vi "AlliGator Compute Smoothed Complex Phasor Array.vi"(8 "error in (no error)":errorcluster, 9 "Time-Gated Reference Decay":cluster{"t Array":dbl[], "I Array":dbl[]}, 10 "Image Array":T17[](array[typedef]), 11 "Sum Image":T17) -> (0 "error out":errorcluster, 1 "Phasor Plot Parameters":T1={"Phasor Frequency"=0.0, "Decay Preprocessing Options & Parameters"={"Background Subtraction Parameters"={"Background Definition Range"={"Min Gate"=0.0, "Max Gate"=0.0}, "Baseline Subtraction Method"=enum."Mean", "Background Subtraction?"=FALSE, "Background File"=path "", "Background Constant"=0.0, "Background Scaling Factor"=1.0, "Background Pile-up Correction"=FALSE, "Background Pixel Well Capacity"=1}, "Decay Preprocessing Parameters"={"Background Subtraction"=FALSE, "Straighten Decay"=FALSE, "Reverse Gates"=FALSE, "1-Normalized Decay"=FALSE, "Smoothen Decay"=FALSE, "Smoothing Parameter"=0.0, "Shift Decay"=FALSE, "Decay Shift Parameters"={"Type"=enum."Default", "Shift"=0.0, "Threshold"=0.0, "Rotate"=FALSE}, "Extrapolate Decay"=FALSE, "Additional Points"=0, "Head Fraction"=0.0, "Pixel-Normalize Decay"=FALSE, "Use Periodicity"=FALSE, "Use Cursors"=FALSE, "Tail Fraction"=0.0, "Use Decay Pre-Processing"=TRUE, "Fold Decay"=FALSE, "# Folds"=1, "[0-1]-Normalized Decay"=FALSE}, "Preprocessing Steps Order"=[]}, "FLI Dataset Modified"=FALSE, "Source Image Settings"={"Low Count Pixels Rejection Options"={"Background Low Threshold Factor"=0.0, "Fixed Low Background Threshold"=0.0, "Reject Low Count Pixels"=FALSE, "Low Percentile"=0.0}, "High Count Pixels Rejection Options"={"Background High Threshold Factor"=0.0, "Fixed High Background Threshold"=20000.0, "Reject High Count Pixels"=FALSE, "High Percentile"=100.0}}, "Data Information"={"Gate Width"=0.0, "Gate Separation"=0.0, "Step (Gate Separation)"=0, "Laser Period"=0.0, "SYNC Period"=0.0, "Channel Name"=0, "Channel Arithmetic"=enum."None", "Pile-up Correction"=FALSE, "Pixel Well Capacity"=1, "Dataset Scaling Factor"=1.0}, "Phasor Plot"={"Phasor Plot Smoothing Options"={"Use Phasor Plot Smoothing"=FALSE, "Kernel Type"=enum."Uniform", "Bin"=1, "Algorithm"=enum."Rapid"}, "Phasor Plot Size"={"H"=0, "V"=0, "Margin"=0.0}, "Selected Image ROI(s)"=FALSE, "All Image ROIs"=FALSE, "Selected Source Image ROI"=0, "Source Image ROIs"=[]}} {"Phasor Plot"."Source Image ROIs"."ROI Descriptor"."Contours"."Type" items=["No Selection", "Point", "Line", "Rectangle", "Oval", "Polygon", "Freehand Region", "Annulus", "Unused2", "Unused3", "Broken Line", "Freehand Line", "Rotated Rectangle"]; "Phasor Plot"."Phasor Plot Smoothing Options"."Bin" min=1 step=2; "Data Information"."Dataset Scaling Factor" min=0.0; "Data Information"."Pixel Well Capacity" min=1 step=1; "Data Information"."Channel Name" items=["Gate"]; "Source Image Settings"."High Count Pixels Rejection Options"."High Percentile" min=0.0 max=100.0; "Source Image Settings"."Low Count Pixels Rejection Options"."Low Percentile" min=0.0 max=100.0; "Decay Preprocessing Options & Parameters"."Decay Preprocessing Parameters"."# Folds" min=1; "Decay Preprocessing Options & Parameters"."Background Subtraction Parameters"."Background Pixel Well Capacity" min=1 step=1}, 2 "Corrected Complex Phasor Array out (VxH)":csg[][](array[numeric]), 3 "Valid Pixel?":bool[][](array[boolean]), 4 "Message":string, 5 "Pre-processed Sum Image (V x H)":sgl[][](array[numeric]), 6 "Phasor Array updated":bool)   [LabVIEW 2021, in "AlliGator Phasor Plot.lvlib"]
doc: "Computes the (smoothed) array of single-pixel phasors."
uses:
  AlliGator Phasor Plot.lvlib
  <vilib>/vision/Image Controls.llb/IMAQ Image.ctl
  AlliGator Phasor Plot Parameters v2.ctl
  Decay Analysis/Decay Preprocessing/AlliGator Decay Preprocessing Options.ctl
  Decay Analysis/Decay Preprocessing/AlliGator Background Subtraction Parameters.ctl
  Decay Analysis/Decay Preprocessing/AlliGator Baseline Subtraction Method.ctl
  Decay Analysis/Decay Preprocessing/AlliGator Decay Preprocessing Parameters.ctl
  Graphs/XY Graph/XY Graph Plot Shift Parameters.ctl
  Graphs/XY Graph/XY Graph Plot Shift Method.ctl
  Settings/AlliGator Low Count Pixels Rejection Options.ctl
  Settings/AlliGator High Count Pixels Rejection Options.ctl
  Settings/AlliGator Gate Arithmetic.ctl
  AlliGator Phasor Plot Smoothing Options.ctl
  Arrays/Kernel Type.ctl
  Arrays/Smoothing Algorithm.ctl
  AlliGator Phasor Plot Size.ctl
  Image/Named ROI Description.ctl
  Globals, Variables, Constants/AlliGator Variables List.ctl
  Settings/AlliGator Pixel Counts Constraints.ctl
  Phasor/Phasor.lvlib
  Decay Analysis/Decay Processing/AlliGator Decay Processing.lvlib
  Globals, Variables, Constants/AlliGator Globals, Variables & Constants.lvlib
  Settings/AlliGator Settings.lvlib
  Decay Analysis/Decay Preprocessing/AlliGator Decay Preprocessing.lvlib
  Graphs/XY Graph/XY Graph Add-Ons.lvlib
  Arrays/Arrays.lvlib
  Image/Image.lvlib
panel:
  # "see the AlliGator License on the block diagram (Ctrl+E or Window:Show Block Diagram)"
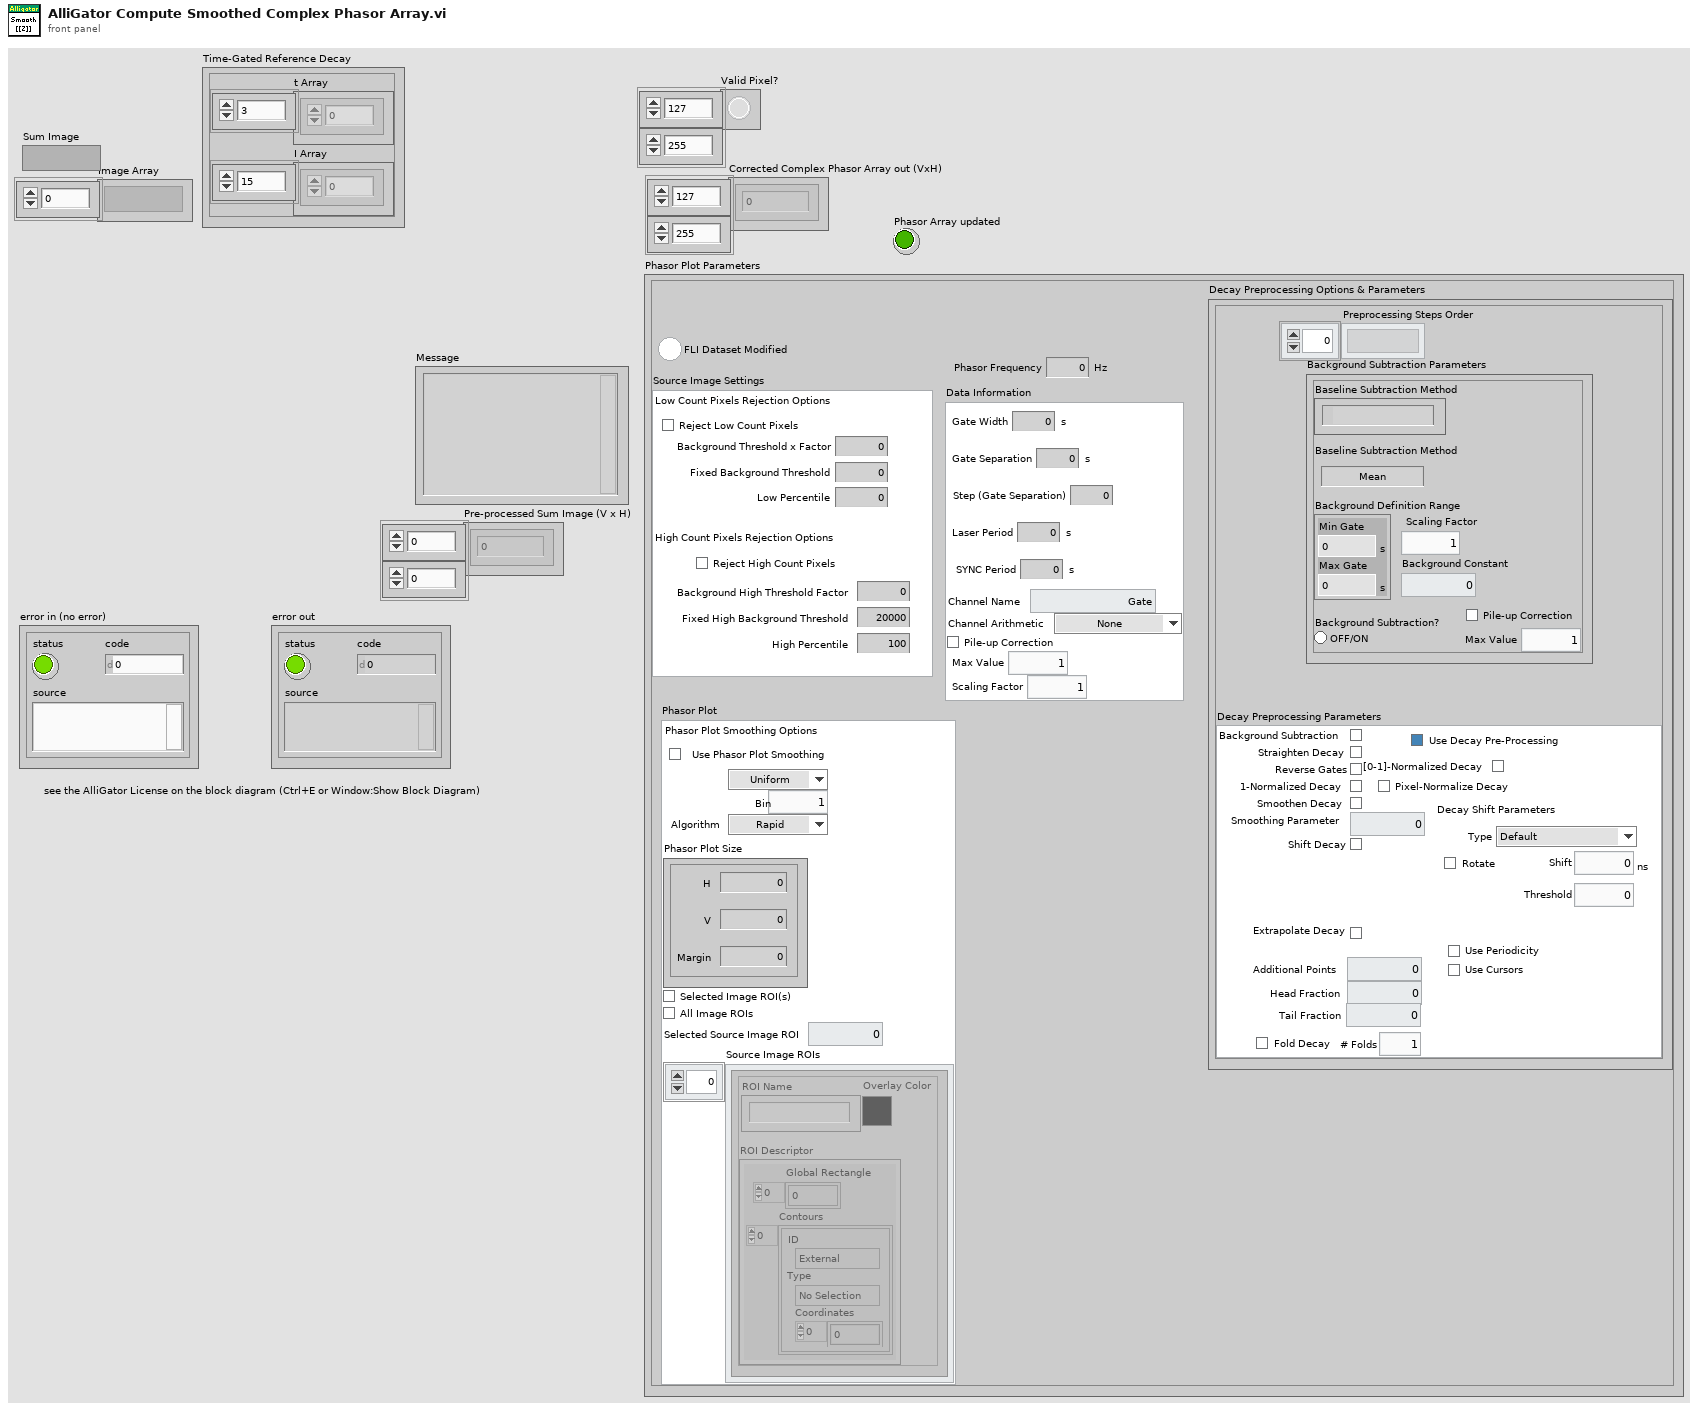
[diagram p1: front panel]
types:
  T1 = typedef "AlliGator Phasor Plot.lvlib/AlliGator Phasor Plot Parameters v2.ctl" = cluster{"Phasor Frequency":dbl[unit], "Decay Preprocessing Options & Parameters":T2, "FLI Dataset Modified":bool, "Source Image Settings":cluster{"Low Count Pixels Rejection Options":T8, "High Count Pixels Rejection Options":T9}, "Data Information":cluster{"Gate Width":dbl[unit], "Gate Separation":dbl[unit], "Step (Gate Separation)":i32, "Laser Period":dbl[unit], "SYNC Period":dbl[unit], "Channel Name":u16, "Channel Arithmetic":T10, "Pile-up Correction":bool, "Pixel Well Capacity":u32, "Dataset Scaling Factor":dbl}, "Phasor Plot":cluster{"Phasor Plot Smoothing Options":T11, "Phasor Plot Size":T14, "Selected Image ROI(s)":bool, "All Image ROIs":bool, "Selected Source Image ROI":i32, "Source Image ROIs":T15[]}}
  T2 = typedef "AlliGator Decay Preprocessing.lvlib/AlliGator Decay Preprocessing Options.ctl" = cluster{"Background Subtraction Parameters":T3, "Decay Preprocessing Parameters":T5, "Preprocessing Steps Order":string[]}
  T3 = typedef "AlliGator Decay Preprocessing.lvlib/AlliGator Background Subtraction Parameters.ctl" = cluster{"Background Definition Range":cluster{"Min Gate":dbl[unit], "Max Gate":dbl[unit]}, "Baseline Subtraction Method":T4, "Background Subtraction?":bool, "Background File":path, "Background Constant":dbl, "Background Scaling Factor":dbl, "Background Pile-up Correction":bool, "Background Pixel Well Capacity":u32}
  T4 = typedef "AlliGator Decay Preprocessing.lvlib/AlliGator Baseline Subtraction Method.ctl" = enum16{"Mean", "Min", "Square Gated Single-Exponential", "File", "Constant"}
  T5 = typedef "AlliGator Decay Preprocessing.lvlib/AlliGator Decay Preprocessing Parameters.ctl" = cluster{"Background Subtraction":bool, "Straighten Decay":bool, "Reverse Gates":bool, "1-Normalized Decay":bool, "Smoothen Decay":bool, "Smoothing Parameter":dbl, "Shift Decay":bool, "Decay Shift Parameters":T6, "Extrapolate Decay":bool, "Additional Points":u32, "Head Fraction":dbl, "Pixel-Normalize Decay":bool, "Use Periodicity":bool, "Use Cursors":bool, "Tail Fraction":dbl, "Use Decay Pre-Processing":bool, "Fold Decay":bool, "# Folds":u32, "[0-1]-Normalized Decay":bool}
  T6 = typedef "XY Graph Add-Ons.lvlib/XY Graph Plot Shift Parameters.ctl" = cluster{"Type":T7, "Shift":dbl[unit], "Threshold":dbl, "Rotate":bool}
  T7 = typedef "XY Graph Add-Ons.lvlib/XY Graph Plot Shift Method.ctl" = enum16{"Default", "CFD", "Threshold", "Cross-Correlation"}
  T8 = typedef "AlliGator Settings.lvlib/AlliGator Low Count Pixels Rejection Options.ctl" = cluster{"Background Low Threshold Factor":dbl, "Fixed Low Background Threshold":dbl, "Reject Low Count Pixels":bool, "Low Percentile":dbl}
  T9 = typedef "AlliGator Settings.lvlib/AlliGator High Count Pixels Rejection Options.ctl" = cluster{"Background High Threshold Factor":dbl, "Fixed High Background Threshold":dbl, "Reject High Count Pixels":bool, "High Percentile":dbl}
  T10 = typedef "AlliGator Settings.lvlib/AlliGator Gate Arithmetic.ctl" = enum16{"None", "INT-G2", "G2/INT*<INT>", "(1 - G2/INT)*<INT>"}
  T11 = typedef "AlliGator Phasor Plot.lvlib/AlliGator Phasor Plot Smoothing Options.ctl" = cluster{"Use Phasor Plot Smoothing":bool, "Kernel Type":T12, "Bin":i32, "Algorithm":T13}
  T12 = typedef "Arrays.lvlib/Kernel Type.ctl" = enum16{"Uniform", "Bilinear", "Gaussian"}
  T13 = typedef "Arrays.lvlib/Smoothing Algorithm.ctl" = enum16{"Rapid", "Thorough"}
  T14 = typedef "AlliGator Phasor Plot.lvlib/AlliGator Phasor Plot Size.ctl" = cluster{"H":i32, "V":i32, "Margin":dbl}
  T15 = typedef "Image.lvlib/Named ROI Description.ctl" = cluster{"ROI Descriptor":T16, "ROI Name":string, "Overlay Color":u32}
  T16 = typedef "ROI Descriptor" = cluster{"Global Rectangle":i32[], "Contours":cluster{"ID":enum32{"External", "Internal"}, "Type":u32, "Coordinates":i32[]}[]}
  T17 = typedef "IMAQ Image.ctl" = refnum<image>
  T18 = typedef "AlliGator Globals, Variables & Constants.lvlib/AlliGator Variables List.ctl" = enum16{"---- GUI ----", "GUI:Initialization Status", "GUI:State Indicators Refnum", "GUI:Original AlliGator Menu Items", "GUI:Current Action Loop State", "GUI:Script in progress", "GUI:Playback", "GUI:Loop Playback", "GUI:Search ROI Used", "GUI:Search ROI", "Decay Graph Max Legend Size", "Intensity Graph Max Legend Size", "Decay Statistics Graph Max Legend Size", "Phasor Graph Max Legend Size", "Phasor Ratio Graph Max Legend Size", "Lifetime Graph Max Legend Size", "---- Files ----", "Files:Export Dataset Frames as Individual Files", "Files:Show Batch Export Help Balloons", "Files:Frames in Dataset", "Files:ptu File Frame Start Indices", "Files:Current Frame in Dataset", "Files:Current Frame Timestamp", "Files:Dataset Loaded", "Files:Dataset Metadata", "Files:Dataset Channel", "Files:Dataset Data Description", "Files:Background Dataset Metadata", "Files:Background Dataset Channel", "Files:Background Dataset Data Description", "Files:Background File Subtraction", "Files:Background File Path", "Files:Background File Pile-up Correction", "Files:Background File Pixel Well Capacity", "Files:Background File Scaling Factor", "Files:Current Dataset Load Settings", "Files:Dataset Path", "Files:ICCD-specific Information", "Files:Macrotime Gate Separation", "------ Python Plugins ------", "Python Plugins:Information", "Python Plugins:Python Session", "Python Plugins:Valid Python Session?", "---- Source Image ----", "Source Image:ROIs", "Source Image:Current ROI", "Source Image:ROI Event Refnum", "X_Source Image:Display Range", "X_Source Image:Palette Information", "X_Source Image:Type of Displayed Image", "X_Time Gate Slider", "Source Image:Palette List", "Source Image:Scale", "Source Image:ROI Overlay Color", "Source Image:Overlay to Erase", "Source Image:Is Displayed Image Accumulated", "Source Image:White Light Image Modified", "Source Image:Mask Image Modified", "---- Image Profile Window ----", "Image Profile:Window Event Refnum", "Image Profile:IntensityType", "Image Profile:Intensity Average Type", "Image Profile:Intensity-weighted SDV", "Image Profile:Box Profile Type", "Image Profile:Window Open", "Image Profile:Plotted Fit Parameter", "------ Phasor Graph -------", "Phasor Graph:Show Line", "---- Phasor Plot ---", "Phasor Plot:Parameters Changed", "Phasor Plot:FLI Dataset Modified since last Calculation", "Phasor Harmonics Data", "Selected Phasor Harmonics", "Phasor Harmonic Manager Event Refnum", "Phasor Plot:ROIs", "Phasor Plot:Current ROI", "Phasor Plot:ROI Event Refnum", "Phasor Plot:Image Reference Points", "Phasor Plot:Computed", "Phasor Plot:Palette Information", "Phasor Plot:Palette List", "Phasor Plot:Phasor Ratio Palette Information", "Phasor Plot:Phasor Ratio Palette List", "Phasor Plot:Image Scale", "Phasor Plot:Image Overlay to Erase", "Phasor Plot:Image Elements to Update", "Phasor Plot:Current Calculation Parameters", "Phasor Plot:Current Calibration Options", "Phasor Plot:Reset Cumulated Phasor Plot", "Phasor Plot:Reference 1", "Phasor Plot:Lifetime Reference 1", "Phasor Plot:Reference 1 Frequency", "Phasor Plot:Reference 2", "Phasor Plot:Lifetime Reference 2", "Phasor Plot:Reference 2 Frequency", "---- Decay Analysis ----", "Number of Selected Decays to Fit", "LS Fit Results", "LAR Fit Results", "BS Fit Results", "Last Decay Max - Min", "Best Fit Parameters", "Best Fit Parameter Names", "Actual Size X", "Actual Size Y", "Binning X", "Binning Y", "Actual # Gates", "Dataset Number", "Gates to...", "Gates Skipped", "Gates to keep", "Gate Step", "Gate Separation", "Reversed Gates", "Pile-up Correction", "Pixel Well Capacity", "Background Subtracted", "Background Subtraction Method", "Background Definition Range", "Background File (deprecated)", "Number of Dataset Accumulated", "Array of Accumulated Dataset Paths", "Do Averaged Datasets", "Destination File Path", "Process Plot Target", "Use 1/D as Phasor Frequency", "---- Decay Fit Parameter Map -----", "Decay Fit Parameter Map:Palette Information", "Decay Fit Parameter Map:Palette List", "Decay Fit Parameter Map:X Resolution", "Decay Fit Parameter Map:Y Resolution", "---- Parameter Map ----", "Parameter Map:Palette Information", "Parameter Map:Palette List", "------- Local Decay Window ---------", "Local Decay Graph Window:Event Refnum", "Local Decay Graph Window:Use normalized IRF for convolution", "----- Miscellaneous ----", "Misc:Skippable Dialog Windows Status"}
  T19 = typedef "AlliGator Settings.lvlib/AlliGator Pixel Counts Constraints.ctl" = cluster{"High Count Pixels Rejection Options":T9, "Low Count Pixels Rejection Options":T8}
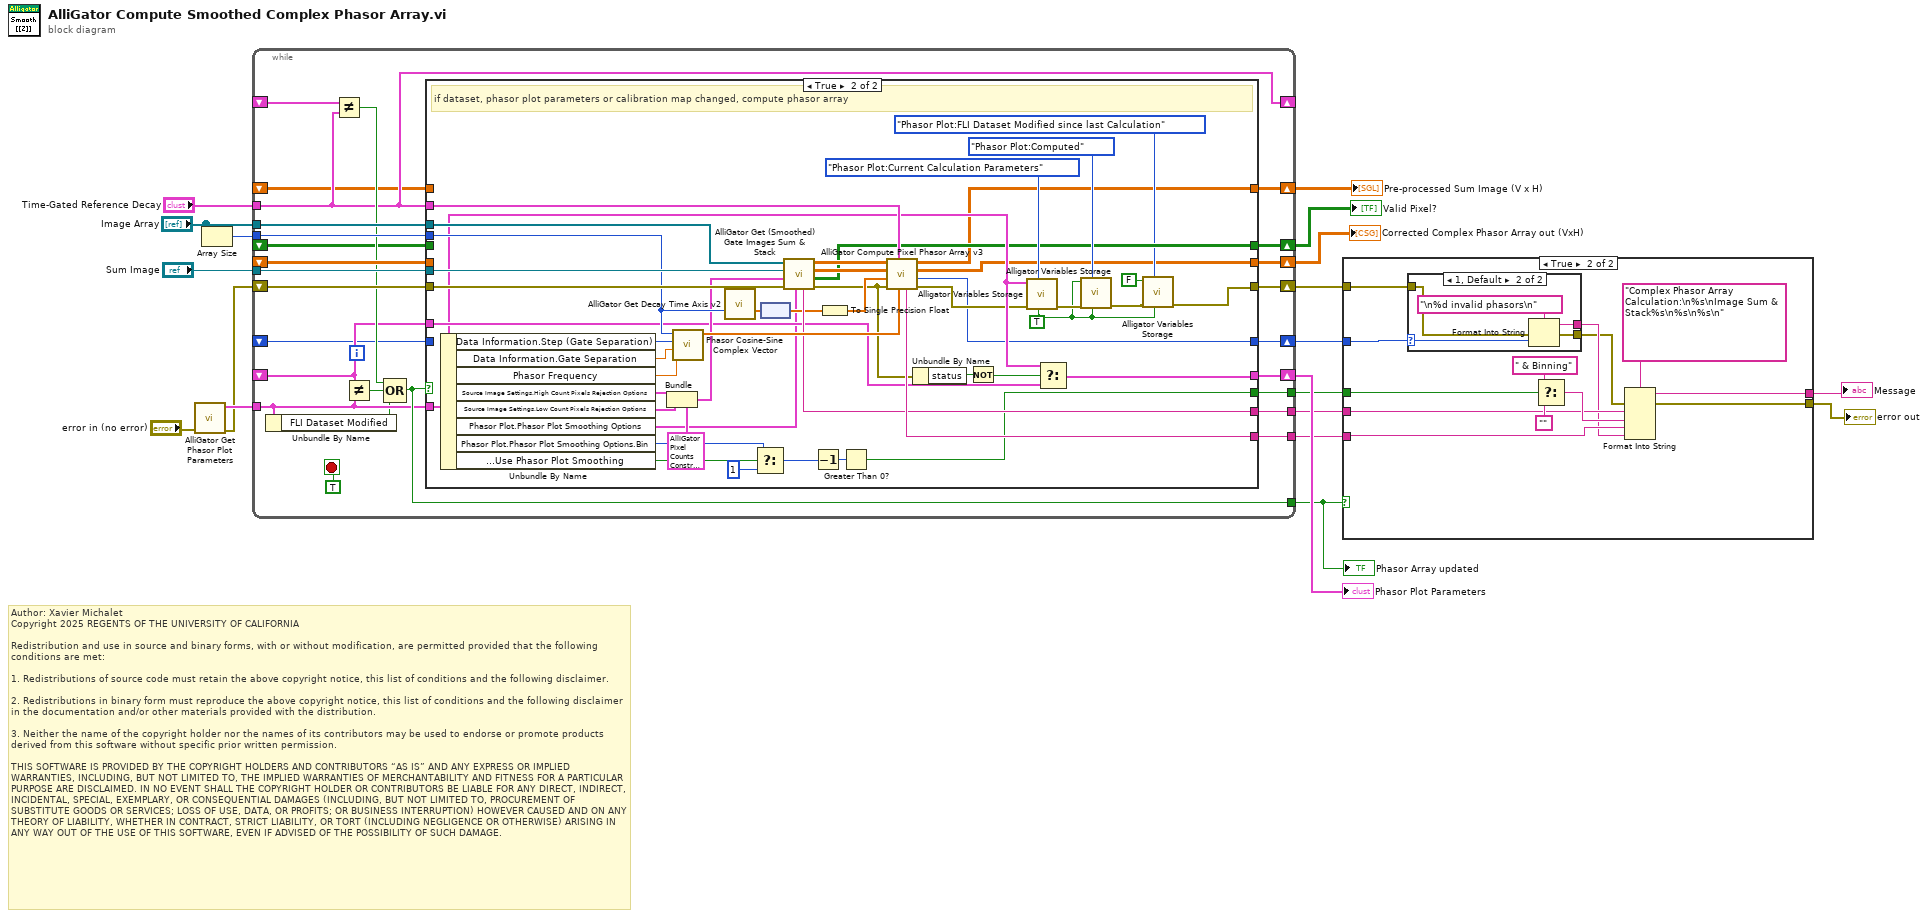
[diagram p0: block diagram]
diagram:
  # "Author: Xavier Michalet\nCopyright 2025 REGENTS OF THE UNIVERSITY OF CALIFORNIA\n\nRedistribution and use in source and binary forms, with or without modification, are permitted provided that the following conditions are met:\n\n1. Redistributions of source code must retain the above copyright notice, this list of conditions and the following disclaimer.\n\n2. Redistributions in binary form must reproduce the above copyright notice, this list of conditions and the following disclaimer in the documentation and/or other materials provided with the distribution.\n\n3. Neither the name of the copyright holder nor the names of its contributors may be used to endorse or promote products derived from this software without specific prior written permission.\n\nTHIS SOFTWARE IS PROVIDED BY THE COPYRIGHT HOLDERS AND CONTRIBUTORS “AS IS” AND ANY EXPRESS OR IMPLIED WARRANTIES, INCLUDING, BUT NOT LIMITED TO, THE IMPLIED WARRANTIES OF MERCHANTABILITY AND FITNESS FOR A PARTICULAR PURPOSE ARE DISCLAIMED. IN NO EVENT SHALL THE COPYRIGHT HOLDER OR CONTRIBUTORS BE LIABLE FOR ANY DIRECT, INDIRECT, INCIDENTAL, SPECIAL, EXEMPLARY, OR CONSEQUENTIAL DAMAGES (INCLUDING, BUT NOT LIMITED TO, PROCUREMENT OF SUBSTITUTE GOODS OR SERVICES; LOSS OF USE, DATA, OR PROFITS; OR BUSINESS INTERRUPTION) HOWEVER CAUSED AND ON ANY THEORY OF LIABILITY, WHETHER IN CONTRACT, STRICT LIABILITY, OR TORT (INCLUDING NEGLIGENCE OR OTHERWISE) ARISING IN ANY WAY OUT OF THE USE OF THIS SOFTWARE, EVEN IF ADVISED OF THE POSSIBILITY OF SUCH DAMAGE."
  n1 = call "AlliGator Get Phasor Plot Parameters.vi"("Error In"="error in (no error)") -> ("Error Out"=w12:errorcluster, "Phasor Plot Parameters"=w16:T1)  [unwired: 8 in, 1 out]
  n2 = Array Size(array="Image Array") -> (size(s)=w15:i32)
  n3 = while {
    tunnel: "Image Array" -> [w44]
    tunnel: "Sum Image" -> [w42]
    tunnel: w16 -> [w23]
    tunnel: w15 -> [w41]
    tunnel: [w40] -> w8
    tunnel: [w38] -> w7
    tunnel: [w37] -> w9
    shift-right: [w39] -> w4
    shift-left: w12 -> [w45]
    shift-right: [w32] -> w11
    shift-left: _ -> [w31]
    shift-right: [w43] -> w18
    shift-left: _ -> [w35]
    tunnel: "Time-Gated Reference Decay" -> [w26]
    shift-right: [w26] -> _
    shift-left: _ -> [w34]
    shift-right: [w30] -> w13
    shift-left: _ -> [w29]
    shift-right: [w28] -> w5
    shift-left: _ -> [w27]
    tunnel: [w24] -> w2
    shift-right: [w21] -> w1
    shift-left: _ -> [w20]
    stop <- TRUE stop-if-true
    n4 = Unbundle By Name(w23) -> ("FLI Dataset Modified"=w22:bool)
    n5 = Not Equal?(x=w34, y=w26) -> (x != y?=w33:bool)
    n6 = Not Equal?(x=w31, y=w23) -> (x != y?=w25:bool)
    n7 = Compound Arithmetic op=OR(w33, w25, w22) -> (w24:bool)
    n8 = case shown="True" w24 {
      tunnel: w45 -> [w50 w97]
      tunnel: w44 -> [_ w95]
      tunnel: [w51 w53] -> w43
      tunnel: w42 -> [_ w88]
      tunnel: w41 -> [_ w87]
      tunnel: [_ w83] -> w40
      tunnel: [w50 w57] -> w39
      tunnel: [_ w82] -> w38
      tunnel: [_ w80] -> w37
      tunnel: w23 -> [_ w73]
      tunnel: w35 -> [w51 _]
      tunnel: w26 -> [_ w78]
      tunnel: [w49 w75] -> w32
      tunnel: w31 -> [w49 w74]
      tunnel: [w48 w68] -> w30
      tunnel: w29 -> [w48 _]
      tunnel: [w47 w64] -> w28
      tunnel: w27 -> [w47 _]
      tunnel: [w46 w52] -> w21
      tunnel: w20 -> [w46 _]
      frame False {
        # "If nothing has changed, do not recompute phasor array"
      }
      frame True {
        w56 = TRUE ("Get(F)/Set")
        # "if dataset, phasor plot parameters or calibration map changed, compute phasor array"
        n9 = Unbundle By Name(w73) -> ("Data Information.Step (Gate Separation)"=w96:i32, "Data Information.Gate Separation"=w92:dbl[unit], "Phasor Frequency"=w89:dbl[unit], "Source Image Settings.High Count Pixels Rejection Options"=w86:T9, "Source Image Settings.Low Count Pixels Rejection Options"=w85:T8, "Phasor Plot.Phasor Plot Smoothing Options"=w59:T11, "Phasor Plot.Phasor Plot Smoothing Options.Bin"=w62:i32, "Phasor Plot.Phasor Plot Smoothing Options.Use Phasor Plot Smoothing"=w63:bool)
        n10 = Bundle(cluster=T19 {"High Count Pixels Rejection Options"={"Background High Threshold Factor"=0.0, "Fixed High Background Threshold"=0.0, "Reject High Count Pixels"=FALSE, "High Percentile"=0.0}, "Low Count Pixels Rejection Options"={"Background Low Threshold Factor"=0.0, "Fixed Low Background Threshold"=0.0, "Reject Low Count Pixels"=FALSE, "Low Percentile"=0.0}} ("Pixel Counts Constraints"), "High Count Pixels Rejection Options"=w86, "Low Count Pixels Rejection Options"=w85) -> (w84:T19)
        n11 = call "Phasor Cosine-Sine Complex Vector.vi"("Phasor Frequency"=w89, "Elementary Gate Separation"=w92, "Step"=w96, "# Gates"=w87) -> ("e^j w t_i Vector"=w91:csg[])  [unwired: 7 in]
        n12 = call "AlliGator Get Decay Time Axis v2.vi"("Number of Gates"=w87) -> ("t Array"=w94:dbl[unit][])  [unwired: 14 in]
        n13 = Select(t=w62, s=w63, f=1) -> (s? t:f=w60:i32)
        n14 = node(w94) -> (w79:dbl[])
        n15 = call "AlliGator Get (Smoothed) Gate Images Sum & Stack.vi"("Phasor Plot Smoothing Options"=w59, "Error In"=w97, "Pixel Counts Constraints"=w84, "Sum Image"=w88, "Image Array"=w95) -> ("Error Out"=w66:errorcluster, "[[Valid Pixel]] VxH Array"=w68:bool[][], "Gate Images Stack (N xV xH)"=w93:sgl[][][], "Sum Image (VxH)"=w90:sgl[][], "Message"=w82:string)  [unwired: 2 in]
        n16 = Decrement(x=w60) -> (x-1=w81:i32)
        n17 = To Single Precision Float(number=w79) -> (single precision float=w67:sgl[])
        n18 = Greater Than 0?(x=w81) -> (x > 0?=w80:bool)
        n19 = call "AlliGator Compute Pixel Phasor Array v3.vi"("e^j w t_i Vector"=w91, "Time-Gated Reference Decay"=w78, "Error In"=w66, "t Array"=w67, "Gate Images Stack (NxVxH)"=w93, "Sum Image (V x H)"=w90) -> ("Error Out"=w65:errorcluster, "# Invalid Phasors"=w64:i32, "Pixel Phasors Array (V x H)"=w53:csg[][], "Pre-processed Sum Image (V x H)"=w52:sgl[][], "Message"=w83:string)  [unwired: 1 in]
        n20 = Unbundle By Name(w66) -> ("status"=w76:bool)
        n21 = Not(x=w76) -> (.not. x?=w72:bool)
        n22 = call "Alligator Variables Storage.vi"("Get(F)/Set"=w56, "AlliGator Variable"=AlliGator_Variables_List."Phasor Plot:Current Calculation Parameters" ("Alligator Variable"), "Error In"=w65, "Data in"=w73) -> ("Error Out"=w71:errorcluster)  [unwired: 5 in, 2 out]
        n23 = Select(t=w73, s=w72, f=w74) -> (s? t:f=w75:T1)
        n24 = call "Alligator Variables Storage.vi"("Get(F)/Set"=w56, "AlliGator Variable"=AlliGator_Variables_List."Phasor Plot:Computed" ("Alligator Variable"), "Error In"=w71, "Data in"=w56) -> ("Error Out"=w58:errorcluster)  [unwired: 5 in, 2 out]
        n25 = call "Alligator Variables Storage.vi"("Get(F)/Set"=w56, "AlliGator Variable"=AlliGator_Variables_List."Phasor Plot:FLI Dataset Modified since last Calculation" ("Alligator Variable"), "Error In"=w58, "Data in"=FALSE ("Get(F)/Set")) -> ("Error Out"=w57:errorcluster)  [unwired: 5 in, 2 out]
      }
    }
  }
  "Corrected Complex Phasor Array out (VxH)" <- w18
  "Valid Pixel?" <- w13
  "Phasor Plot Parameters" <- w11
  "Phasor Array updated" <- w2
  "Pre-processed Sum Image (V x H)" <- w1
  n26 = case shown="True" w2 {
    tunnel: w9 -> [_ w109]
    tunnel: w8 -> [_ w106]
    tunnel: w7 -> [_ w105]
    tunnel: [_ w104] -> w6
    tunnel: w5 -> [_ w103]
    tunnel: w4 -> [w98 w101]
    tunnel: [w98 w99] -> w3
    frame False {
    }
    frame True {
      n27 = case shown="1, Default" w103 {
        selector: w103 -> [_ w117]
        tunnel: w101 -> [w112 w116]
        tunnel: [w112 w115] -> w100
        tunnel: [_ w113] -> w102
        frame 0 {
        }
        frame 1, Default {
          n28 = Format Into String(format string="\n%d invalid phasors\n", error in=w116, w117) -> (resulting string=w113:string, error out=w115:errorcluster)  [unwired: 1 in]
        }
      }
      n29 = Select(t=" & Binning" ("input 1"), s=w109, f="") -> (s? t:f=w107:string)
      n30 = Format Into String(format string="Complex Phasor Array Calculation:\n%s\nImage Sum & Stack%s\n%s\n%s\n", error in=w100, w105, w107, w106, w102) -> (resulting string=w104:string, error out=w99:errorcluster)  [unwired: 1 in]
    }
  }
  "error out" <- w3
  "Message" <- w6
